vi "Ball Intake Calibrations.vi"() -> ()   [LabVIEW 2016]
panel:
  in  "Ball Intake Calibrations File Location":path=path "C:/ni-rt/startup/BallIntakeCalibrations.txt"
  out "Intake Reverse Speed (throttle)":dbl
  out "Intake Forward Speed (throttle)":dbl
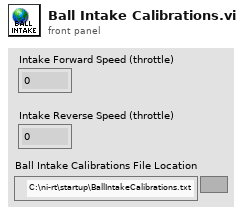
[diagram p1: front panel]
diagram:
